vi "Close OPC UA Client.vi"(8 "error in (no error)":errorcluster, 11 "OPC UA Client.lvclass":refnum<class "OPC UA Client.lvclass">) -> (0 "error out":errorcluster)   [LabVIEW 2016, in "OPC UA Client.lvclass"]
uses:
  OPC UA Client.lvclass
  OPC UA Client.lvclass/OPC UA Client.ctl
  <vilib>/OPCUA/NI OPC UA Client.lvlib
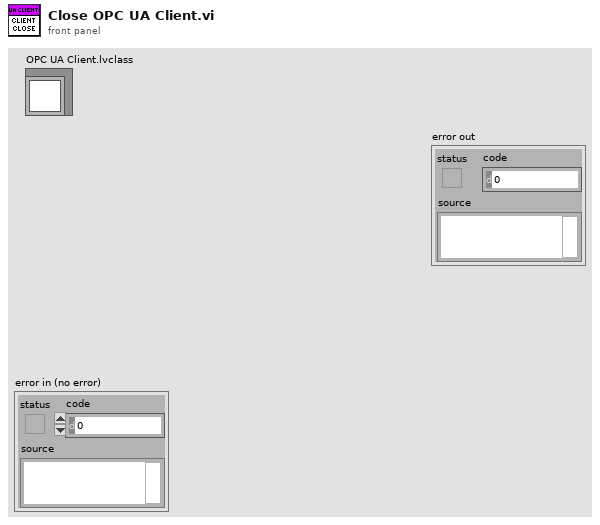
[diagram p1: front panel]
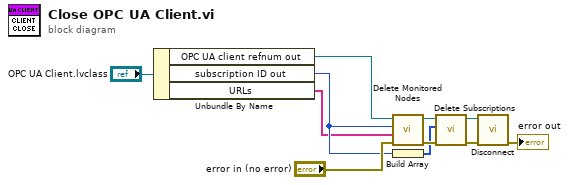
[diagram p0: block diagram]
diagram:
  n1 = Unbundle By Name("OPC UA Client.lvclass") -> ("OPC UA client refnum out"=w3:refnum<k21>, "subscription ID out"=w2:u32, "URLs"=w1:string[])
  n2 = call <vilib>:"Delete Monitored Nodes.vi"("error in (no error)"="error in (no error)", "array of node path"=w1, "subscription ID in"=w2, "OPC UA client refnum in"=w3) -> ("error out"=w10:errorcluster, "OPC UA client refnum out"=w11:refnum<k21>)  [unwired: 4 in, 2 out]
  n3 = Build Array(w2) -> (w7:u32[])
  n4 = call <vilib>:"Delete Subscriptions.vi"("error in (no error)"=w10, "array of subscription ID"=w7, "OPC UA client refnum in"=w11) -> ("error out"=w8:errorcluster, "OPC UA client refnum out"=w9:refnum<k21>)  [unwired: 6 in, 1 out]
  n5 = call <vilib>:"Disconnect.vi"("error in (no error)"=w8, "OPC UA client refnum in"=w9) -> ("error out"=→"error out":errorcluster)  [unwired: 9 in]
